vi "HandleObservationSync.vi"(8 "error in (no error)":errorcluster, 11 "S4GUI in":refnum<class "S4GUI.lvclass">) -> (0 "error out":errorcluster, 3 "S4GUI out":refnum<class "S4GUI.lvclass">)   [LabVIEW 2018, in "S4GUI.lvclass"] (continued)
            tunnel: w4132 -> [w4190 w4209]
            tunnel: [w4188 w4208] -> w4134
            tunnel: w4135 -> [w4189 _]
            tunnel: w4129 -> [w4187 _]
            frame False {
              n1517 = case shown="0, Default" w4187 {
                selector: w4187 -> [_ w4204]
                tunnel: [w4191 w4199] -> w4188
                tunnel: w4190 -> [w4194 w4205]
                tunnel: w4189 -> [w4193 _]
                frame 0, Default {
                  n1518 = disable-structure shown="Enabled" {
                    disable-tunnel: w4193 -> [w4196 w4197]
                    disable-tunnel: [w4195 w4197] -> w4192
                    frame Disabled {
                      # "Verifica o incremento \ndo CyclesDone simultaneamente"
                      n1519 = Increment(x=w4196) -> (x+1=w4195:u32)
                    }
                    frame Enabled {
                      # "OV20241106:\nNão verifica mais o CyclesDone\nem 327 enquanto espera o ACTIVE\nem 326."
                    }
                  }
                  n1520 = Bundle By Name(cluster=w4194, "Obs_state"=w4192) -> (w4191:refnum<class "S4GUI.lvclass">)
                }
                frame 1..15 {
                  n1521 = Number To Decimal String(number=w4204) -> (decimal integer string=w4201:string)  [unwired: 1 in]
                  n1522 = Concatenate Strings("CHANNEL ERROR <", w4201, ">: Error flag TRUE - see ACS panel.  HandleObservationSync.vi - state 326.") -> (w4203:string)
                  n1523 = Bundle By Name(cluster=w4205, "Obs_state"=u32 1, "Error Msg"=w4203) -> (w4199:refnum<class "S4GUI.lvclass">)
                }
              }
            }
            frame True {
              # "ACTIVE detectado.\nIniciou aquisição..."
              n1524 = Tick Count (ms)() -> (millisecond timer value=w4206:u32)
              n1525 = local write "time307"(w4206) -> ()
              n1526 = Bundle By Name(cluster=w4209, "Obs_state"=u32 328) -> (w4208:refnum<class "S4GUI.lvclass">)
            }
          }
          n1527 = Bundle By Name(cluster=w4134, "mode EXPOSE"=w4137) -> (w4181:refnum<class "S4GUI.lvclass">)
        }
        frame 327 {
          # "T= canais receberam STOP"
          n1528 = Unbundle By Name(w4333) -> ("cyclesDone"=w4328:u32)
          n1529 = call-dynamic "Read AcquisitionA.vi"("error in (no error)"=w4366, "S4ACS_GUI in"=w4333) -> ("error out"=w4348:errorcluster, "Acquisition.lvclass"=w4349:refnum<class "Acquisition.lvclass">, "S4ACS_GUI out"=w4368:refnum<class "S4GUI.lvclass">)  [unwired: 7 in]
          n1530 = call-dynamic "Read enabled.vi"("error in (no error)"=w4348, "Server in"=w4349) -> ("error out"=w4347:errorcluster, "enabled"=w4324:bool, "Server out"=w4346:refnum<class "Acquisition.lvclass">)  [unwired: 7 in]
          n1531 = case shown="True" w4324 {
            tunnel: w4347 -> [w4522 w4539]
            tunnel: [w4523 w4537] -> w4369
            tunnel: [w4522 w4536] -> w4367
            tunnel: [0 ("State") w4532] -> w4319
            tunnel: w4346 -> [w4523 w4531]
            tunnel: w4328 -> [_ w4530]
            tunnel: [TRUE w4529] -> w4332
            tunnel: [FALSE ("stopping") w4525] -> w4315
            frame False {
            }
            frame True {
              n1532 = call-dynamic "Read Channel.vi"("error in (no error)"=w4539, "Acquisition in"=w4531) -> ("error out"=w4535:errorcluster, "Channel.lvclass"=w4534:refnum<class "Channel.lvclass">, "Acquisition out"=w4538:refnum<class "Acquisition.lvclass">)  [unwired: 7 in]
              n1533 = call-dynamic "Read CyclesDone.vi"("error in (no error)"=w4535, "Channel in"=w4534) -> ("error out"=w4527:errorcluster, "CyclesDone"=w4532:u32, "Channel out"=w4533:refnum<class "Channel.lvclass">)  [unwired: 7 in]
              n1534 = Increment(x=w4530) -> (x+1=w4524:u32)
              n1535 = Equal?(x=w4532, y=w4524) -> (x = y?=w4529:bool)
              n1536 = call-dynamic "Read stopping.vi"("error in (no error)"=w4527, "Channel in"=w4533) -> ("error out"=w4526:errorcluster, "stopping"=w4525:bool, "Channel out"=w4528:refnum<class "Channel.lvclass">)  [unwired: 7 in]
              n1537 = call-dynamic "Write Channel.vi"("error in (no error)"=w4526, "Channel.lvclass"=w4528, "Acquisition in"=w4538) -> ("error out"=w4536:errorcluster, "Acquisition out"=w4537:refnum<class "Acquisition.lvclass">)  [unwired: 7 in]
            }
          }
          n1538 = call-dynamic "Write AcquisitionA.vi"("error in (no error)"=w4367, "Acquisition.lvclass"=w4369, "S4ACS_GUI in"=w4368) -> ("error out"=w4364:errorcluster, "S4ACS_GUI out"=w4363:refnum<class "S4GUI.lvclass">)  [unwired: 7 in]
          n1539 = call "Read AcquisitionB.vi"("error in (no error)"=w4364, "S4ACS_GUI in"=w4363) -> ("error out"=w4342:errorcluster, "Acquisition.lvclass"=w4345:refnum<class "Acquisition.lvclass">, "S4ACS_GUI out"=w4365:refnum<class "S4GUI.lvclass">)  [unwired: 7 in]
          n1540 = call-dynamic "Read enabled.vi"("error in (no error)"=w4342, "Server in"=w4345) -> ("error out"=w4343:errorcluster, "enabled"=w4323:bool, "Server out"=w4344:refnum<class "Acquisition.lvclass">)  [unwired: 7 in]
          n1541 = case shown="True" w4323 {
            tunnel: w4343 -> [w4501 w4518]
            tunnel: w4344 -> [w4502 w4517]
            tunnel: [0 ("State") w4510] -> w4318
            tunnel: [w4501 w4516] -> w4362
            tunnel: [w4502 w4515] -> w4361
            tunnel: w4328 -> [_ w4509]
            tunnel: [TRUE w4508] -> w4329
            tunnel: [FALSE ("stopping") w4504] -> w4314
            frame False {
            }
            frame True {
              n1542 = call-dynamic "Read Channel.vi"("error in (no error)"=w4518, "Acquisition in"=w4517) -> ("error out"=w4513:errorcluster, "Channel.lvclass"=w4514:refnum<class "Channel.lvclass">, "Acquisition out"=w4511:refnum<class "Acquisition.lvclass">)  [unwired: 7 in]
              n1543 = call-dynamic "Read CyclesDone.vi"("error in (no error)"=w4513, "Channel in"=w4514) -> ("error out"=w4506:errorcluster, "CyclesDone"=w4510:u32, "Channel out"=w4512:refnum<class "Channel.lvclass">)  [unwired: 7 in]
              n1544 = Increment(x=w4509) -> (x+1=w4503:u32)
              n1545 = Equal?(x=w4510, y=w4503) -> (x = y?=w4508:bool)
              n1546 = call-dynamic "Read stopping.vi"("error in (no error)"=w4506, "Channel in"=w4512) -> ("error out"=w4505:errorcluster, "stopping"=w4504:bool, "Channel out"=w4507:refnum<class "Channel.lvclass">)  [unwired: 7 in]
              n1547 = call-dynamic "Write Channel.vi"("error in (no error)"=w4505, "Channel.lvclass"=w4507, "Acquisition in"=w4511) -> ("error out"=w4516:errorcluster, "Acquisition out"=w4515:refnum<class "Acquisition.lvclass">)  [unwired: 7 in]
            }
          }
          n1548 = Max & Min(x=w4319, y=w4318) -> (max(x,y)=w4331:u32)  [unwired: 1 out]
          n1549 = call "Write AcquisitionB.vi"("error in (no error)"=w4362, "Acquisition.lvclass"=w4361, "S4ACS_GUI in"=w4365) -> ("error out"=w4354:errorcluster, "S4ACS_GUI out"=w4353:refnum<class "S4GUI.lvclass">)  [unwired: 7 in]
          n1550 = call-dynamic "Read AcquisitionC.vi"("error in (no error)"=w4354, "S4ACS_GUI in"=w4353) -> ("error out"=w4339:errorcluster, "Acquisition.lvclass"=w4341:refnum<class "Acquisition.lvclass">, "S4ACS_GUI out"=w4356:refnum<class "S4GUI.lvclass">)  [unwired: 7 in]
          n1551 = call-dynamic "Read enabled.vi"("error in (no error)"=w4339, "Server in"=w4341) -> ("error out"=w4338:errorcluster, "enabled"=w4322:bool, "Server out"=w4340:refnum<class "Acquisition.lvclass">)  [unwired: 7 in]
          n1552 = case shown="True" w4322 {
            tunnel: [w4480 w4497] -> w4357
            tunnel: [w4481 w4496] -> w4355
            tunnel: w4338 -> [w4480 w4493]
            tunnel: w4340 -> [w4481 w4494]
            tunnel: [0 ("State") w4492] -> w4317
            tunnel: w4328 -> [_ w4491]
            tunnel: [TRUE w4490] -> w4327
            tunnel: [FALSE ("stopping") w4483] -> w4313
            frame False {
            }
            frame True {
              n1553 = call-dynamic "Read Channel.vi"("error in (no error)"=w4493, "Acquisition in"=w4494) -> ("error out"=w4489:errorcluster, "Channel.lvclass"=w4488:refnum<class "Channel.lvclass">, "Acquisition out"=w4495:refnum<class "Acquisition.lvclass">)  [unwired: 7 in]
              n1554 = call-dynamic "Read CyclesDone.vi"("error in (no error)"=w4489, "Channel in"=w4488) -> ("error out"=w4485:errorcluster, "CyclesDone"=w4492:u32, "Channel out"=w4487:refnum<class "Channel.lvclass">)  [unwired: 7 in]
              n1555 = Increment(x=w4491) -> (x+1=w4482:u32)
              n1556 = Equal?(x=w4492, y=w4482) -> (x = y?=w4490:bool)
              n1557 = call-dynamic "Read stopping.vi"("error in (no error)"=w4485, "Channel in"=w4487) -> ("error out"=w4484:errorcluster, "stopping"=w4483:bool, "Channel out"=w4486:refnum<class "Channel.lvclass">)  [unwired: 7 in]
              n1558 = call-dynamic "Write Channel.vi"("error in (no error)"=w4484, "Channel.lvclass"=w4486, "Acquisition in"=w4495) -> ("error out"=w4497:errorcluster, "Acquisition out"=w4496:refnum<class "Acquisition.lvclass">)  [unwired: 7 in]
            }
          }
          n1559 = call-dynamic "Write AcquisitionC.vi"("error in (no error)"=w4357, "Acquisition.lvclass"=w4355, "S4ACS_GUI in"=w4356) -> ("error out"=w4351:errorcluster, "S4ACS_GUI out"=w4352:refnum<class "S4GUI.lvclass">)  [unwired: 7 in]
          n1560 = call-dynamic "Read AcquisitionD.vi"("error in (no error)"=w4351, "S4ACS_GUI in"=w4352) -> ("error out"=w4335:errorcluster, "Acquisition.lvclass"=w4337:refnum<class "Acquisition.lvclass">, "S4ACS_GUI out"=w4358:refnum<class "S4GUI.lvclass">)  [unwired: 7 in]
          n1561 = call-dynamic "Read enabled.vi"("error in (no error)"=w4335, "Server in"=w4337) -> ("error out"=w4334:errorcluster, "enabled"=w4325:bool, "Server out"=w4336:refnum<class "Acquisition.lvclass">)  [unwired: 7 in]
          n1562 = case shown="True" w4325 {
            tunnel: [w4460 w4476] -> w4360
            tunnel: [w4459 w4475] -> w4359
            tunnel: w4336 -> [w4460 w4474]
            tunnel: w4334 -> [w4459 w4473]
            tunnel: [0 ("State") w4471] -> w4316
            tunnel: w4328 -> [_ w4470]
            tunnel: [TRUE w4469] -> w4326
            tunnel: [FALSE ("stopping") w4462] -> w4312
            frame False {
            }
            frame True {
              n1563 = call-dynamic "Read Channel.vi"("error in (no error)"=w4473, "Acquisition in"=w4474) -> ("error out"=w4468:errorcluster, "Channel.lvclass"=w4467:refnum<class "Channel.lvclass">, "Acquisition out"=w4472:refnum<class "Acquisition.lvclass">)  [unwired: 7 in]
              n1564 = call-dynamic "Read CyclesDone.vi"("error in (no error)"=w4468, "Channel in"=w4467) -> ("error out"=w4464:errorcluster, "CyclesDone"=w4471:u32, "Channel out"=w4466:refnum<class "Channel.lvclass">)  [unwired: 7 in]
              n1565 = Increment(x=w4470) -> (x+1=w4461:u32)
              n1566 = Equal?(x=w4471, y=w4461) -> (x = y?=w4469:bool)
              n1567 = call-dynamic "Read stopping.vi"("error in (no error)"=w4464, "Channel in"=w4466) -> ("error out"=w4463:errorcluster, "stopping"=w4462:bool, "Channel out"=w4465:refnum<class "Channel.lvclass">)  [unwired: 7 in]
              n1568 = call-dynamic "Write Channel.vi"("error in (no error)"=w4463, "Channel.lvclass"=w4465, "Acquisition in"=w4472) -> ("error out"=w4475:errorcluster, "Acquisition out"=w4476:refnum<class "Acquisition.lvclass">)  [unwired: 7 in]
            }
          }
          n1569 = Build Array(w4324, w4323, w4322, w4325) -> (w4321:bool[])
          n1570 = Boolean Array To Number(Boolean array=w4321) -> (number=w4320:u32)
          n1571 = Max & Min(x=w4317, y=w4316) -> (max(x,y)=w4330:u32)  [unwired: 1 out]
          n1572 = Compound Arithmetic op=AND(w4332, w4329, w4327, w4326) -> (w4311:bool)
          n1573 = case shown="15" w4320 {
            tunnel: w4319 -> [w4412 _ w4424 _ w4433 _ w4439 w4445 _ w4451 w4454 _]
            tunnel: w4316 -> [w4411 w4415 w4420 w4427 w4428 w4436 w4438 _ _ _ _ _]
            tunnel: w4318 -> [w4410 w4413 _ _ w4432 w4434 _ w4444 w4448 _ w4453 _]
            tunnel: w4317 -> [w4409 w4414 w4419 w4425 _ _ _ w4443 w4447 w4450 _ _]
            tunnel: [w4405 w4416 w4421 w4426 w4429 w4435 w4437 w4440 w4446 w4449 w4452 TRUE] -> _
            frame 15 {
              # "A,B,C,D ativos"
              n1574 = Equal?(x=w4412, y=w4410) -> (x = y?=w4408:bool)
              n1575 = Equal?(x=w4409, y=w4411) -> (x = y?=w4406:bool)
              n1576 = Equal?(x=w4410, y=w4409) -> (x = y?=w4407:bool)
              n1577 = Compound Arithmetic op=AND(w4408, w4407, w4406) -> (w4405:bool)
            }
            frame 14 {
              # "B,C e,D ativos"
              n1578 = Equal?(x=w4413, y=w4414) -> (x = y?=w4418:bool)
              n1579 = Equal?(x=w4414, y=w4415) -> (x = y?=w4417:bool)
              n1580 = Compound Arithmetic op=AND(w4418, w4417) -> (w4416:bool)
            }
            frame 13 {
              # "A,C e,D ativos"
              n1581 = Equal?(x=w4424, y=w4419) -> (x = y?=w4423:bool)
              n1582 = Equal?(x=w4419, y=w4420) -> (x = y?=w4422:bool)
              n1583 = Compound Arithmetic op=AND(w4423, w4422) -> (w4421:bool)
            }
            frame 12 {
              # "Só C e D ativos"
              n1584 = Equal?(x=w4425, y=w4427) -> (x = y?=w4426:bool)
            }
            frame 11 {
              # "A,B e,D ativos"
              n1585 = Equal?(x=w4433, y=w4432) -> (x = y?=w4431:bool)
              n1586 = Equal?(x=w4432, y=w4428) -> (x = y?=w4430:bool)
              n1587 = Compound Arithmetic op=AND(w4431, w4430) -> (w4429:bool)
            }
            frame 10 {
              # "Só B e D ativos"
              n1588 = Equal?(x=w4434, y=w4436) -> (x = y?=w4435:bool)
            }
            frame 9 {
              # "Só A e D ativos"
              n1589 = Equal?(x=w4439, y=w4438) -> (x = y?=w4437:bool)
            }
            frame 7 {
              # "A,B,C ativos"
              n1590 = Equal?(x=w4445, y=w4444) -> (x = y?=w4442:bool)
              n1591 = Equal?(x=w4444, y=w4443) -> (x = y?=w4441:bool)
              n1592 = Compound Arithmetic op=AND(w4442, w4441) -> (w4440:bool)
            }
            frame 6 {
              # "Só B e C ativos"
              n1593 = Equal?(x=w4448, y=w4447) -> (x = y?=w4446:bool)
            }
            frame 5 {
              # "Só A e C ativos"
              n1594 = Equal?(x=w4451, y=w4450) -> (x = y?=w4449:bool)
            }
            frame 3 {
              # "só A e B ativos"
              n1595 = Equal?(x=w4454, y=w4453) -> (x = y?=w4452:bool)
            }
            frame 0..2, 4, 8, Default {
              # "nenhum ou só 1  \ncanal ativo."
            }
          }
          n1596 = Max & Min(x=w4331, y=w4330) -> (max(x,y)=w4309:u32)  [unwired: 1 out]
          n1597 = Compound Arithmetic op=OR(w4315, w4314, w4313, w4312) -> (w4310:bool)
          n1598 = call-dynamic "Write AcquisitionD.vi"("error in (no error)"=w4359, "Acquisition.lvclass"=w4360, "S4ACS_GUI in"=w4358) -> ("error out"=w4350:errorcluster, "S4ACS_GUI out"=w4307:refnum<class "S4GUI.lvclass">)  [unwired: 7 in]
          n1599 = case shown="False" w4311 {
            tunnel: w4307 -> [w4372 w4393]
            tunnel: [w4378 w4392] -> w4306
            tunnel: w4310 -> [_ w4394]
            tunnel: w4309 -> [_ w4391]
            tunnel: w4308 -> [w4370 w4390]
            frame False {
              # "Aguardando iniciar exposição por 5s"
              n1600 = local read "time1"() -> (w4371:u32)
              n1601 = Tick Count (ms)() -> (millisecond timer value=w4377:u32)
              n1602 = Subtract(x=w4377, y=w4371) -> (x-y=w4374:u32)
              n1603 = To Double Precision Float(number=w4374) -> (double precision float=w4376:dbl)
              n1604 = Less?(x=5000.0 ("y"), y=w4376) -> (x < y?=w4375:bool)
              n1605 = case shown="True" w4375 {
                tunnel: w4372 -> [w4382 w4389]
                tunnel: [w4381 w4388] -> w4378
                tunnel: w4370 -> [w4380 _]
                frame False {
                  n1606 = disable-structure shown="Enabled" {
                    disable-tunnel: w4380 -> [w4384 w4385]
                    disable-tunnel: [w4383 w4385] -> w4379
                    frame Disabled {
                      # "Volta para esperar ACTIVE."
                      n1607 = Decrement(x=w4384) -> (x-1=w4383:u32)
                    }
                    frame Enabled {
                    }
                  }
                  n1608 = Bundle By Name(cluster=w4382, "Obs_state"=w4379) -> (w4381:refnum<class "S4GUI.lvclass">)
                }
                frame True {
                  n1609 = Bundle By Name(cluster=w4389, "Obs_state"=u32 1, "Error Msg"="ERROR: Init Acquisition Timeout. HandleObservationSync.vi - state 327.") -> (w4388:refnum<class "S4GUI.lvclass">)
                }
              }
            }
            frame True {
              # "STOP?"
              # "CIclo Avançou."
              n1610 = case shown="False" w4394 {
                tunnel: w4393 -> [w4398 w4404]
                tunnel: [w4397 w4403] -> w4392
                tunnel: w4391 -> [w4396 w4402]
                tunnel: w4390 -> [_ w4401]
                frame True {
                  # "STOP acionado."
                  n1611 = Bundle By Name(cluster=w4398, "Obs_state"=u32 0, "cyclesDone"=w4396) -> (w4397:refnum<class "S4GUI.lvclass">)
                }
                frame False {
                  # "Vai verificar fim dos ciclos"
                  n1612 = Increment(x=w4401) -> (x+1=w4400:u32)
                  n1613 = Increment(x=w4400) -> (x+1=w4399:u32)
                  n1614 = Bundle By Name(cluster=w4404, "Obs_state"=w4399, "cyclesDone"=w4402) -> (w4403:refnum<class "S4GUI.lvclass">)
                }
              }
            }
          }
        }
        frame 328 {
          # "T= canais receberam STOP"
          n1615 = Unbundle By Name(w4564) -> ("cyclesDone"=w4558:u32)
          n1616 = call-dynamic "Read AcquisitionA.vi"("error in (no error)"=w4600, "S4ACS_GUI in"=w4564) -> ("error out"=w4579:errorcluster, "Acquisition.lvclass"=w4580:refnum<class "Acquisition.lvclass">, "S4ACS_GUI out"=w4602:refnum<class "S4GUI.lvclass">)  [unwired: 7 in]
          n1617 = call-dynamic "Read enabled.vi"("error in (no error)"=w4579, "Server in"=w4580) -> ("error out"=w4578:errorcluster, "enabled"=w4554:bool, "Server out"=w4577:refnum<class "Acquisition.lvclass">)  [unwired: 7 in]
          n1618 = case shown="False" w4554 {
            tunnel: w4578 -> [w4751 w4768]
            tunnel: [w4752 w4766] -> w4603
            tunnel: [w4751 w4765] -> w4601
            tunnel: [0 ("State") w4761] -> w4549
            tunnel: w4577 -> [w4752 w4760]
            tunnel: w4558 -> [_ w4759]
            tunnel: [TRUE w4758] -> w4563
            tunnel: [FALSE ("stopping") w4754] -> w4545
            frame False {
            }
            frame True {
              n1619 = call-dynamic "Read Channel.vi"("error in (no error)"=w4768, "Acquisition in"=w4760) -> ("error out"=w4764:errorcluster, "Channel.lvclass"=w4763:refnum<class "Channel.lvclass">, "Acquisition out"=w4767:refnum<class "Acquisition.lvclass">)  [unwired: 7 in]
              n1620 = call-dynamic "Read CyclesDone.vi"("error in (no error)"=w4764, "Channel in"=w4763) -> ("error out"=w4756:errorcluster, "CyclesDone"=w4761:u32, "Channel out"=w4762:refnum<class "Channel.lvclass">)  [unwired: 7 in]
              n1621 = Increment(x=w4759) -> (x+1=w4753:u32)
              n1622 = Equal?(x=w4761, y=w4753) -> (x = y?=w4758:bool)
              n1623 = call-dynamic "Read stopping.vi"("error in (no error)"=w4756, "Channel in"=w4762) -> ("error out"=w4755:errorcluster, "stopping"=w4754:bool, "Channel out"=w4757:refnum<class "Channel.lvclass">)  [unwired: 7 in]
              n1624 = call-dynamic "Write Channel.vi"("error in (no error)"=w4755, "Channel.lvclass"=w4757, "Acquisition in"=w4767) -> ("error out"=w4765:errorcluster, "Acquisition out"=w4766:refnum<class "Acquisition.lvclass">)  [unwired: 7 in]
            }
          }
          n1625 = call-dynamic "Write AcquisitionA.vi"("error in (no error)"=w4601, "Acquisition.lvclass"=w4603, "S4ACS_GUI in"=w4602) -> ("error out"=w4596:errorcluster, "S4ACS_GUI out"=w4595:refnum<class "S4GUI.lvclass">)  [unwired: 7 in]
          n1626 = call "Read AcquisitionB.vi"("error in (no error)"=w4596, "S4ACS_GUI in"=w4595) -> ("error out"=w4573:errorcluster, "Acquisition.lvclass"=w4576:refnum<class "Acquisition.lvclass">, "S4ACS_GUI out"=w4597:refnum<class "S4GUI.lvclass">)  [unwired: 7 in]
          n1627 = call-dynamic "Read enabled.vi"("error in (no error)"=w4573, "Server in"=w4576) -> ("error out"=w4574:errorcluster, "enabled"=w4553:bool, "Server out"=w4575:refnum<class "Acquisition.lvclass">)  [unwired: 7 in]
          n1628 = case shown="True" w4553 {
            tunnel: w4574 -> [w4730 w4747]
            tunnel: w4575 -> [w4731 w4746]
            tunnel: [0 ("State") w4739] -> w4548
            tunnel: [w4730 w4745] -> w4594
            tunnel: [w4731 w4744] -> w4593
            tunnel: w4558 -> [_ w4738]
            tunnel: [TRUE w4737] -> w4559
            tunnel: [FALSE ("stopping") w4733] -> w4544
            frame False {
            }
            frame True {
              n1629 = call-dynamic "Read Channel.vi"("error in (no error)"=w4747, "Acquisition in"=w4746) -> ("error out"=w4742:errorcluster, "Channel.lvclass"=w4743:refnum<class "Channel.lvclass">, "Acquisition out"=w4740:refnum<class "Acquisition.lvclass">)  [unwired: 7 in]
              n1630 = call-dynamic "Read CyclesDone.vi"("error in (no error)"=w4742, "Channel in"=w4743) -> ("error out"=w4735:errorcluster, "CyclesDone"=w4739:u32, "Channel out"=w4741:refnum<class "Channel.lvclass">)  [unwired: 7 in]
              n1631 = Increment(x=w4738) -> (x+1=w4732:u32)
              n1632 = Equal?(x=w4739, y=w4732) -> (x = y?=w4737:bool)
              n1633 = call-dynamic "Read stopping.vi"("error in (no error)"=w4735, "Channel in"=w4741) -> ("error out"=w4734:errorcluster, "stopping"=w4733:bool, "Channel out"=w4736:refnum<class "Channel.lvclass">)  [unwired: 7 in]
              n1634 = call-dynamic "Write Channel.vi"("error in (no error)"=w4734, "Channel.lvclass"=w4736, "Acquisition in"=w4740) -> ("error out"=w4745:errorcluster, "Acquisition out"=w4744:refnum<class "Acquisition.lvclass">)  [unwired: 7 in]
            }
          }
          n1635 = Max & Min(x=w4549, y=w4548) -> (max(x,y)=w4562:u32)  [unwired: 1 out]
          n1636 = call "Write AcquisitionB.vi"("error in (no error)"=w4594, "Acquisition.lvclass"=w4593, "S4ACS_GUI in"=w4597) -> ("error out"=w4586:errorcluster, "S4ACS_GUI out"=w4585:refnum<class "S4GUI.lvclass">)  [unwired: 7 in]
          n1637 = call-dynamic "Read AcquisitionC.vi"("error in (no error)"=w4586, "S4ACS_GUI in"=w4585) -> ("error out"=w4570:errorcluster, "Acquisition.lvclass"=w4572:refnum<class "Acquisition.lvclass">, "S4ACS_GUI out"=w4588:refnum<class "S4GUI.lvclass">)  [unwired: 7 in]
          n1638 = call-dynamic "Read enabled.vi"("error in (no error)"=w4570, "Server in"=w4572) -> ("error out"=w4569:errorcluster, "enabled"=w4552:bool, "Server out"=w4571:refnum<class "Acquisition.lvclass">)  [unwired: 7 in]
          n1639 = case shown="False" w4552 {
            tunnel: [w4709 w4726] -> w4589
            tunnel: [w4710 w4725] -> w4587
            tunnel: w4569 -> [w4709 w4722]
            tunnel: w4571 -> [w4710 w4723]
            tunnel: [0 ("State") w4721] -> w4547
            tunnel: w4558 -> [_ w4720]
            tunnel: [TRUE w4719] -> w4557
            tunnel: [FALSE ("stopping") w4712] -> w4543
            frame False {
            }
            frame True {
              n1640 = call-dynamic "Read Channel.vi"("error in (no error)"=w4722, "Acquisition in"=w4723) -> ("error out"=w4718:errorcluster, "Channel.lvclass"=w4717:refnum<class "Channel.lvclass">, "Acquisition out"=w4724:refnum<class "Acquisition.lvclass">)  [unwired: 7 in]
              n1641 = call-dynamic "Read CyclesDone.vi"("error in (no error)"=w4718, "Channel in"=w4717) -> ("error out"=w4714:errorcluster, "CyclesDone"=w4721:u32, "Channel out"=w4716:refnum<class "Channel.lvclass">)  [unwired: 7 in]
              n1642 = Increment(x=w4720) -> (x+1=w4711:u32)
              n1643 = Equal?(x=w4721, y=w4711) -> (x = y?=w4719:bool)
              n1644 = call-dynamic "Read stopping.vi"("error in (no error)"=w4714, "Channel in"=w4716) -> ("error out"=w4713:errorcluster, "stopping"=w4712:bool, "Channel out"=w4715:refnum<class "Channel.lvclass">)  [unwired: 7 in]
              n1645 = call-dynamic "Write Channel.vi"("error in (no error)"=w4713, "Channel.lvclass"=w4715, "Acquisition in"=w4724) -> ("error out"=w4726:errorcluster, "Acquisition out"=w4725:refnum<class "Acquisition.lvclass">)  [unwired: 7 in]
            }
          }
          n1646 = call-dynamic "Write AcquisitionC.vi"("error in (no error)"=w4589, "Acquisition.lvclass"=w4587, "S4ACS_GUI in"=w4588) -> ("error out"=w4583:errorcluster, "S4ACS_GUI out"=w4584:refnum<class "S4GUI.lvclass">)  [unwired: 7 in]
          n1647 = call-dynamic "Read AcquisitionD.vi"("error in (no error)"=w4583, "S4ACS_GUI in"=w4584) -> ("error out"=w4566:errorcluster, "Acquisition.lvclass"=w4568:refnum<class "Acquisition.lvclass">, "S4ACS_GUI out"=w4590:refnum<class "S4GUI.lvclass">)  [unwired: 7 in]
          n1648 = call-dynamic "Read enabled.vi"("error in (no error)"=w4566, "Server in"=w4568) -> ("error out"=w4565:errorcluster, "enabled"=w4555:bool, "Server out"=w4567:refnum<class "Acquisition.lvclass">)  [unwired: 7 in]
          n1649 = case shown="True" w4555 {
            tunnel: [w4689 w4705] -> w4592
            tunnel: [w4688 w4704] -> w4591
            tunnel: w4567 -> [w4689 w4703]
            tunnel: w4565 -> [w4688 w4702]
            tunnel: [0 ("State") w4700] -> w4546
            tunnel: w4558 -> [_ w4699]
            tunnel: [TRUE w4698] -> w4556
            tunnel: [FALSE ("stopping") w4691] -> w4542
            frame False {
            }
            frame True {
              n1650 = call-dynamic "Read Channel.vi"("error in (no error)"=w4702, "Acquisition in"=w4703) -> ("error out"=w4697:errorcluster, "Channel.lvclass"=w4696:refnum<class "Channel.lvclass">, "Acquisition out"=w4701:refnum<class "Acquisition.lvclass">)  [unwired: 7 in]
              n1651 = call-dynamic "Read CyclesDone.vi"("error in (no error)"=w4697, "Channel in"=w4696) -> ("error out"=w4693:errorcluster, "CyclesDone"=w4700:u32, "Channel out"=w4695:refnum<class "Channel.lvclass">)  [unwired: 7 in]
              n1652 = Increment(x=w4699) -> (x+1=w4690:u32)
              n1653 = Equal?(x=w4700, y=w4690) -> (x = y?=w4698:bool)
              n1654 = call-dynamic "Read stopping.vi"("error in (no error)"=w4693, "Channel in"=w4695) -> ("error out"=w4692:errorcluster, "stopping"=w4691:bool, "Channel out"=w4694:refnum<class "Channel.lvclass">)  [unwired: 7 in]
              n1655 = call-dynamic "Write Channel.vi"("error in (no error)"=w4692, "Channel.lvclass"=w4694, "Acquisition in"=w4701) -> ("error out"=w4704:errorcluster, "Acquisition out"=w4705:refnum<class "Acquisition.lvclass">)  [unwired: 7 in]
            }
          }
          n1656 = Build Array(w4554, w4553, w4552, w4555) -> (w4551:bool[])
          n1657 = Boolean Array To Number(Boolean array=w4551) -> (number=w4550:u32)
          n1658 = Max & Min(x=w4547, y=w4546) -> (max(x,y)=w4561:u32)  [unwired: 1 out]
          n1659 = Compound Arithmetic op=AND(w4563, w4559, w4557, w4556) -> (w4540:bool)
          n1660 = case shown="15" w4550 {
            tunnel: w4549 -> [w4611 _ w4623 _ w4632 _ w4638 w4644 _ w4650 w4653 _]
            tunnel: w4546 -> [w4610 w4614 w4619 w4626 w4627 w4635 w4637 _ _ _ _ _]
            tunnel: w4548 -> [w4609 w4612 _ _ w4631 w4633 _ w4643 w4647 _ w4652 _]
            tunnel: w4547 -> [w4608 w4613 w4618 w4624 _ _ _ w4642 w4646 w4649 _ _]
            tunnel: [w4604 w4615 w4620 w4625 w4628 w4634 w4636 w4639 w4645 w4648 w4651 TRUE] -> _
            frame 15 {
              # "A,B,C,D ativos"
              n1661 = Equal?(x=w4611, y=w4609) -> (x = y?=w4607:bool)
              n1662 = Equal?(x=w4608, y=w4610) -> (x = y?=w4605:bool)
              n1663 = Equal?(x=w4609, y=w4608) -> (x = y?=w4606:bool)
              n1664 = Compound Arithmetic op=AND(w4607, w4606, w4605) -> (w4604:bool)
            }
            frame 14 {
              # "B,C e,D ativos"
              n1665 = Equal?(x=w4612, y=w4613) -> (x = y?=w4617:bool)
              n1666 = Equal?(x=w4613, y=w4614) -> (x = y?=w4616:bool)
              n1667 = Compound Arithmetic op=AND(w4617, w4616) -> (w4615:bool)
            }
            frame 13 {
              # "A,C e,D ativos"
              n1668 = Equal?(x=w4623, y=w4618) -> (x = y?=w4622:bool)
              n1669 = Equal?(x=w4618, y=w4619) -> (x = y?=w4621:bool)
              n1670 = Compound Arithmetic op=AND(w4622, w4621) -> (w4620:bool)
            }
            frame 12 {
              # "Só C e D ativos"
              n1671 = Equal?(x=w4624, y=w4626) -> (x = y?=w4625:bool)
            }
            frame 11 {
              # "A,B e,D ativos"
              n1672 = Equal?(x=w4632, y=w4631) -> (x = y?=w4630:bool)
              n1673 = Equal?(x=w4631, y=w4627) -> (x = y?=w4629:bool)
              n1674 = Compound Arithmetic op=AND(w4630, w4629) -> (w4628:bool)
            }
            frame 10 {
              # "Só B e D ativos"
              n1675 = Equal?(x=w4633, y=w4635) -> (x = y?=w4634:bool)
            }
            frame 9 {
              # "Só A e D ativos"
              n1676 = Equal?(x=w4638, y=w4637) -> (x = y?=w4636:bool)
            }
            frame 7 {
              # "A,B,C ativos"
              n1677 = Equal?(x=w4644, y=w4643) -> (x = y?=w4641:bool)
              n1678 = Equal?(x=w4643, y=w4642) -> (x = y?=w4640:bool)
              n1679 = Compound Arithmetic op=AND(w4641, w4640) -> (w4639:bool)
            }
            frame 6 {
              # "Só B e C ativos"
              n1680 = Equal?(x=w4647, y=w4646) -> (x = y?=w4645:bool)
            }
            frame 5 {
              # "Só A e C ativos"
              n1681 = Equal?(x=w4650, y=w4649) -> (x = y?=w4648:bool)
            }
            frame 3 {
              # "só A e B ativos"
              n1682 = Equal?(x=w4653, y=w4652) -> (x = y?=w4651:bool)
            }
            frame 0..2, 4, 8, Default {
              # "nenhum ou só 1  \ncanal ativo."
            }
          }
          n1683 = Max & Min(x=w4562, y=w4561) -> (max(x,y)=w4560:u32)  [unwired: 1 out]
          n1684 = Compound Arithmetic op=OR(w4545, w4544, w4543, w4542) -> (w4541:bool)
          n1685 = call-dynamic "Write AcquisitionD.vi"("error in (no error)"=w4591, "Acquisition.lvclass"=w4592, "S4ACS_GUI in"=w4590) -> ("error out"=w4581:errorcluster, "S4ACS_GUI out"=w4582:refnum<class "S4GUI.lvclass">)  [unwired: 7 in]
          n1686 = case shown="False" w4540 {
            tunnel: w4582 -> [w4665 w4675]
            tunnel: [w4664 w4674] -> w4599
            tunnel: w4598 -> [_ w4673]
            tunnel: w4560 -> [_ w4672]
            tunnel: w4541 -> [_ w4671]
            frame False {
              # "Aguardando avanço do ciclo."
              n1687 = local read "time307"() -> (w4655:u32)
              n1688 = Tick Count (ms)() -> (millisecond timer value=w4663:u32)
              n1689 = Subtract(x=w4663, y=w4655) -> (x-y=w4660:u32)
              n1690 = call-dynamic "GetGreatestCube.vi"("S4GUI in"=w4665) -> ("S4GUI out"=w4656:refnum<class "S4GUI.lvclass">, "greatest (ms)"=w4658:dbl)  [unwired: 8 in, 1 out]
              n1691 = To Double Precision Float(number=w4660) -> (double precision float=w4662:dbl)
              n1692 = Add(x=5000.0 ("y"), y=w4658) -> (x+y=w4657:dbl)
              n1693 = Less?(x=w4657, y=w4662) -> (x < y?=w4661:bool)
              n1694 = case shown="False" w4661 {
                tunnel: w4656 -> [w4666 w4670]
                tunnel: [w4666 w4669] -> w4664
                frame False {
                }
                frame True {
                  n1695 = Bundle By Name(cluster=w4670, "Obs_state"=u32 1, "Error Msg"="ERROR: Acquisition Timeout. HandleObservationSync.vi - state 328.") -> (w4669:refnum<class "S4GUI.lvclass">)
                }
              }
            }
            frame True {
              # "Ciclo avançou."
              # "STOP?"
              n1696 = case shown="False" w4671 {
                tunnel: w4675 -> [w4679 w4684]
                tunnel: [w4678 w4683] -> w4674
                tunnel: w4673 -> [_ w4681]
                tunnel: w4672 -> [w4677 w4680]
                frame True {
                  n1697 = Bundle By Name(cluster=w4679, "Obs_state"=u32 0, "cyclesDone"=w4677) -> (w4678:refnum<class "S4GUI.lvclass">)
                }
                frame False {
                  n1698 = Increment(x=w4681) -> (x+1=w4682:u32)
                  n1699 = Bundle By Name(cluster=w4684, "Obs_state"=w4682, "cyclesDone"=w4680) -> (w4683:refnum<class "S4GUI.lvclass">)
                }
              }
            }
          }
        }
        frame 329 {
          n1700 = disable-structure shown="Enabled" {
            disable-tunnel: w4773 -> [w4787 w4793]
            disable-tunnel: w4772 -> [w4786 w4800]
            disable-tunnel: [w4785 w4800] -> w4771
            disable-tunnel: [w4783 w4801] -> w4770
            disable-tunnel: w4769 -> [_ w4794]
            frame Disabled {
              n1701 = call-dynamic "Read ciclos.vi"("error in (no error)"=w4786, "S4ACS_GUI in"=w4787) -> ("error out"=w4775:errorcluster, "ciclos"=w4780:u32, "S4ACS_GUI out"=w4788:refnum<class "S4GUI.lvclass">)  [unwired: 7 in]
              n1702 = Decrement(x=w4780) -> (x-1=w4774:u32)
              n1703 = Greater Than 0?(x=w4774) -> (x > 0?=w4781:bool)
              n1704 = case shown="False" w4781 {
                selector: w4781 -> [w4790 w4792]
                tunnel: w4774 -> [_ w4791]
                tunnel: [w4790 w4792] -> w4779
                tunnel: [u32 0 w4791] -> w4776
                frame False {
                }
                frame True {
                }
              }
              n1705 = Select(t=u32 323, s=w4779, f=u32 0) -> (s? t:f=w4782:u32)
              n1706 = call-dynamic "Write ciclos.vi"("error in (no error)"=w4775, "ciclos"=w4776, "S4ACS_GUI in"=w4788) -> ("error out"=w4785:errorcluster, "S4ACS_GUI out"=w4784:refnum<class "S4GUI.lvclass">)  [unwired: 7 in]
              n1707 = Bundle By Name(cluster=w4784, "Obs_state"=w4782) -> (w4783:refnum<class "S4GUI.lvclass">)
            }
            frame Enabled {
              n1708 = Unbundle By Name(w4793) -> ("TotalCiclos"=w4803:u32, "cyclesDone"=w4802:u32)
              n1709 = Subtract(x=w4803, y=w4802) -> (x-y=w4796:u32)
              n1710 = Greater Than 0?(x=w4796) -> (x > 0?=w4799:bool)
              n1711 = disable-structure shown="Enabled" {
                disable-tunnel: [w4805 u32 325 ("t")] -> w4795
                disable-tunnel: w4794 -> [w4804 _]
                frame Disabled {
                  n1712 = Increment(x=w4804) -> (x+1=w4805:u32)
                }
                frame Enabled {
                }
              }
              n1713 = Select(t=w4795, s=w4799, f=u32 0) -> (s? t:f=w4798:u32)
              n1714 = Bundle By Name(cluster=w4793, "ciclos"=w4796, "Obs_state"=w4798) -> (w4801:refnum<class "S4GUI.lvclass">)
            }
          }
        }
        frame 350 {
          n1715 = flat-sequence {
            tunnel: w4808 -> [w4848]
            tunnel: [w4848] -> w4807
            frame #0 {
              n1716 = Tick Count (ms)() -> (millisecond timer value=→"timer350":u32)
            }
          }
          n1717 = call "Read Instrument.lvclass.vi"("error in (no error)"=w4807, "S4ACS_GUI in"=w4843) -> ("error out"=w4846:errorcluster, "Instrument.lvclass"=w4847:refnum<class "Instrument.lvclass">, "S4ACS_GUI out"=w4844:refnum<class "S4GUI.lvclass">)  [unwired: 7 in]
          n1718 = call "Read WPROT.vi"("error in (no error)"=w4846, "Instrument in"=w4847) -> ("error out"=w4836:errorcluster, "Opt_Selector.lvclass"=w4837:refnum<class "Opt_Selector.lvclass">, "Instrument out"=w4845:refnum<class "Instrument.lvclass">)  [unwired: 7 in]
          n1719 = call-dynamic "getTargetPos.vi"("error in (no error)"=w4836, "Opt_Selector in"=w4837) -> ("error out"=w4835:errorcluster, "Target Pos"=w4815:u16, "Opt_Selector out"=w4834:refnum<class "Opt_Selector.lvclass">)  [unwired: 7 in]
          n1720 = Build Array(-1.0 ("element"), 0.0 ("element"), 22.5 ("element"), 45.0 ("element"), 67.5 ("element"), 90.0 ("element"), 112.5 ("element"), 135.0 ("element"), 157.5 ("element"), 180.0 ("element"), 202.5 ("element"), 225.0 ("element"), 247.5 ("element"), 270.0 ("element"), 292.5 ("element"), 315.0 ("element"), 337.5 ("element")) -> (w4827:dbl[])
          n1721 = Index Array(array=w4827, index=w4815) -> (element=w4814:dbl)
          n1722 = case shown="0, Default" w4815 {
            selector: w4815 -> [_ w4877]
            tunnel: w4845 -> [w4857 w4865]
            tunnel: [w4857 w4865] -> w4810
            tunnel: [w4854 w4864] -> w4809
            tunnel: w4840 -> [_ w4879]
            tunnel: [u32 352 w4878] -> w4839
            tunnel: w4835 -> [w4855 w4873]
            tunnel: w4834 -> [w4856 w4872]
            tunnel: w4814 -> [_ w4867]
            tunnel: [w4852 w4866] -> w4811
            frame 0, Default {
              # "Terminou uma sequência.\nRecupera as posições em SEQ e desvia para 311 para verificar se há mais ciclos."
              # "Recupera a sequencia anterior para o caso \nde repetição da sequencia (sem precisar clicar \nnas posicoes desejadas novamente)."
              n1723 = call-dynamic "Read sequencia_ant.vi"("error in (no error)"=w4855, "Opt_Selector in"=w4856) -> ("error out"=w4851:errorcluster, "sequencia_ant"=w4850:u16, "Opt_Selector out"=w4853:refnum<class "Opt_Selector.lvclass">)  [unwired: 7 in]
              n1724 = call-dynamic "Write sequencia.vi"("error in (no error)"=w4851, "sequencia"=w4850, "Opt_Selector in"=w4853) -> ("error out"=w4854:errorcluster, "Opt_Selector out"=w4852:refnum<class "Opt_Selector.lvclass">)  [unwired: 7 in]
            }
            frame 1..16 {
              # "Espera até 40 x 0.25s (= 10s) para\nmecanismo entrar em READY"
              n1725 = Number To Decimal String(number=w4877) -> (decimal integer string=w4876:string)  [unwired: 1 in]
              n1726 = Concatenate Strings("WP" ("string"), w4876) -> (w4874:string)
              n1727 = call "Write target name.vi"("error in (no error)"=w4873, "target name"=w4874, "Optics in"=w4872) -> ("error out"=w4870:errorcluster, "Optics out"=w4871:refnum<class "Opt_Selector.lvclass">)  [unwired: 7 in]
              n1728 = call "Write target.vi"("error in (no error)"=w4870, "target"=w4867, "Optics in"=w4871) -> ("error out"=w4869:errorcluster, "Optics out"=w4868:refnum<class "Opt_Selector.lvclass">)  [unwired: 7 in]
              n1729 = call-dynamic "Read State Machine.vi"("error in (no error)"=w4869, "Device in"=w4868) -> ("error out"=w4881:errorcluster, "State Machine.lvclass"=w4883:refnum<class "State Machine.lvclass">, "Device out"=w4880:refnum<class "Opt_Selector.lvclass">)  [unwired: 7 in]
              n1730 = Increment(x=w4879) -> (x+1=w4878:u32)
              n1731 = call "Next State.vi"("error in (no error)"=w4881, "New_State"=1, "State Machine in"=w4883) -> ("error out"=w4861:errorcluster, "State Machine out"=w4863:refnum<class "State Machine.lvclass">)  [unwired: 7 in]
              n1732 = call-dynamic "Write Timer.vi"("error in (no error)"=w4861, "Timer"=u32 40, "State Machine in"=w4863) -> ("error out"=w4860:errorcluster, "State Machine out"=w4862:refnum<class "State Machine.lvclass">)  [unwired: 7 in]
              n1733 = call-dynamic "Write State Machine.vi"("error in (no error)"=w4860, "State Machine.lvclass"=w4862, "Device in"=w4880) -> ("error out"=w4864:errorcluster, "Device out"=w4866:refnum<class "Opt_Selector.lvclass">)  [unwired: 7 in]
            }
          }
          n1734 = call "Write WPROT.vi"("error in (no error)"=w4809, "Opt_Selector.lvclass"=w4811, "Instrument in"=w4810) -> ("error out"=w4813:errorcluster, "Instrument out"=w4812:refnum<class "Instrument.lvclass">)  [unwired: 7 in]
          n1735 = call "Write Instrument.lvclass.vi"("error in (no error)"=w4813, "Instrument.lvclass"=w4812, "S4ACS_GUI in"=w4844) -> ("error out"=w4842:errorcluster, "S4ACS_GUI out"=w4841:refnum<class "S4GUI.lvclass">)  [unwired: 7 in]
          n1736 = Bundle By Name(cluster=w4841, "Obs_state"=w4839) -> (w4838:refnum<class "S4GUI.lvclass">)
        }
        frame 351 {
          # "Espera terminar o movimento da lamina para disparar a aquisição\ndos canais ativos.\n\nOV 20230424: Não precisa mais atualizar o valor de WPPOS com o\ncomando WRITE_HEADER porque o ACS já recebeu a sequência de\nposições da lâmina."
          n1737 = flat-sequence {
            tunnel: w4894 -> [w4913]
            tunnel: [w4913] -> w4893
            frame #0 {
              n1738 = Tick Count (ms)() -> (millisecond timer value=w4912:u32)
              "timer351" <- w4912
              n1739 = local read "time1"() -> (w4911:u32)
              n1740 = Subtract(x=w4912, y=w4911) -> (x-y=→"delay wp 2":u32)
            }
          }
          n1741 = call "Read Instrument.lvclass.vi"("error in (no error)"=w4893, "S4ACS_GUI in"=w4903) -> ("error out"=w4908:errorcluster, "Instrument.lvclass"=w4909:refnum<class "Instrument.lvclass">, "S4ACS_GUI out"=w4905:refnum<class "S4GUI.lvclass">)  [unwired: 7 in]
          n1742 = call "Read WPROT.vi"("error in (no error)"=w4908, "Instrument in"=w4909) -> ("error out"=w4900:errorcluster, "Opt_Selector.lvclass"=w4899:refnum<class "Opt_Selector.lvclass">, "Instrument out"=w4907:refnum<class "Instrument.lvclass">)  [unwired: 7 in]
          n1743 = call-dynamic "Read State Machine.vi"("error in (no error)"=w4900, "Device in"=w4899) -> ("error out"=w4901:errorcluster, "State Machine.lvclass"=w4902:refnum<class "State Machine.lvclass">, "Device out"=w4897:refnum<class "Opt_Selector.lvclass">)  [unwired: 7 in]
          n1744 = call-dynamic "Read State.vi"("error in (no error)"=w4901, "State Machine in"=w4902) -> ("error out"=w4891:errorcluster, "State"=w4895:i32, "State Machine out"=w4892:refnum<class "State Machine.lvclass">)  [unwired: 7 in]
          n1745 = Equal To 0?(x=w4895) -> (x = 0?=w4886:bool)
          n1746 = call-dynamic "Write State Machine.vi"("error in (no error)"=w4891, "State Machine.lvclass"=w4892, "Device in"=w4897) -> ("error out"=w4896:errorcluster, "Device out"=w4898:refnum<class "Opt_Selector.lvclass">)  [unwired: 7 in]
          n1747 = call "Write WPROT.vi"("error in (no error)"=w4896, "Opt_Selector.lvclass"=w4898, "Instrument in"=w4907) -> ("error out"=w4904:errorcluster, "Instrument out"=w4906:refnum<class "Instrument.lvclass">)  [unwired: 7 in]
          n1748 = call "Write Instrument.lvclass.vi"("error in (no error)"=w4904, "Instrument.lvclass"=w4906, "S4ACS_GUI in"=w4905) -> ("error out"=w4884:errorcluster, "S4ACS_GUI out"=w4887:refnum<class "S4GUI.lvclass">)  [unwired: 7 in]
          n1749 = Select(t=u32 350, s=w4886, f=w4885) -> (s? t:f=w4890:u32)
          n1750 = Bundle By Name(cluster=w4887, "Obs_state"=w4890) -> (w4888:refnum<class "S4GUI.lvclass">)
        }
        frame 352 {
          n1751 = disable-structure shown="Enabled" {
            disable-tunnel: w4917 -> [w4931 w4944]
            disable-tunnel: w4916 -> [w4930 w4942]
            disable-tunnel: [w4929 w4942] -> w4915
            disable-tunnel: [w4927 w4943] -> w4914
            frame Disabled {
              n1752 = call-dynamic "Read ciclos.vi"("error in (no error)"=w4930, "S4ACS_GUI in"=w4931) -> ("error out"=w4919:errorcluster, "ciclos"=w4924:u32, "S4ACS_GUI out"=w4932:refnum<class "S4GUI.lvclass">)  [unwired: 7 in]
              n1753 = Decrement(x=w4924) -> (x-1=w4918:u32)
              n1754 = Greater Than 0?(x=w4918) -> (x > 0?=w4925:bool)
              n1755 = case shown="False" w4925 {
                selector: w4925 -> [w4934 w4936]
                tunnel: w4918 -> [_ w4935]
                tunnel: [w4934 w4936] -> w4923
                tunnel: [u32 0 w4935] -> w4920
                frame False {
                }
                frame True {
                }
              }
              n1756 = Select(t=u32 323, s=w4923, f=u32 0) -> (s? t:f=w4926:u32)
              n1757 = call-dynamic "Write ciclos.vi"("error in (no error)"=w4919, "ciclos"=w4920, "S4ACS_GUI in"=w4932) -> ("error out"=w4929:errorcluster, "S4ACS_GUI out"=w4928:refnum<class "S4GUI.lvclass">)  [unwired: 7 in]
              n1758 = Bundle By Name(cluster=w4928, "Obs_state"=w4926) -> (w4927:refnum<class "S4GUI.lvclass">)
            }
            frame Enabled {
              n1759 = Unbundle By Name(w4944) -> ("cycles wprot"=w4945:u32)
              n1760 = Decrement(x=w4945) -> (x-1=w4937:u32)
              n1761 = Greater Than 0?(x=w4937) -> (x > 0?=w4941:bool)
              n1762 = Select(t=u32 350, s=w4941, f=u32 0) -> (s? t:f=w4940:u32)
              n1763 = Bundle By Name(cluster=w4944, "Obs_state"=w4940, "cycles wprot"=w4937) -> (w4943:refnum<class "S4GUI.lvclass">)
            }
          }
        }
        frame 360 {
          w4946 = u32 0 ("cyclesDone")
          # "Inicia o Ticks com\nvalor do relogio atual"
          # "Espera até 40 x 0.25s (= 10s) para\nmecanismo entrar em READY"
          # "Busca próximo valor de foco..."
          n1764 = flat-sequence {
            tunnel: w4963 -> [w4978]
            tunnel: [w4978] -> w4962
            frame #0 {
              n1765 = Tick Count (ms)() -> (millisecond timer value=→"time7":u32)
            }
          }
          n1766 = call-dynamic "Read TelFocus.lvclass.vi"("error in (no error)"=w4962, "S4GUI in"=w4974) -> ("error out"=w4976:errorcluster, "TelFocus.lvclass"=w4977:refnum<class "TelFocus.lvclass">, "S4GUI out"=w4975:refnum<class "S4GUI.lvclass">)  [unwired: 7 in]
          n1767 = call-dynamic "GetNextFocus.vi"("error in (no error)"=w4976, "TelFocus in"=w4977) -> ("error out"=w4960:errorcluster, "TelFocus out"=w4961:refnum<class "TelFocus.lvclass">)  [unwired: 8 in]
          n1768 = call-dynamic "Read SecMirror.lvclass.vi"("error in (no error)"=w4960, "TelFocus in"=w4961) -> ("error out"=w4947:errorcluster, "SecMirror.lvclass"=w4948:refnum<class "SecMirror.lvclass">, "TelFocus out"=w4965:refnum<class "TelFocus.lvclass">)  [unwired: 7 in]
          n1769 = call-dynamic "Read State Machine.vi"("error in (no error)"=w4947, "Device in"=w4948) -> ("error out"=w4957:errorcluster, "State Machine.lvclass"=w4959:refnum<class "State Machine.lvclass">, "Device out"=w4956:refnum<class "SecMirror.lvclass">)  [unwired: 7 in]
          n1770 = call "Next State.vi"("error in (no error)"=w4957, "New_State"=1, "State Machine in"=w4959) -> ("error out"=w4954:errorcluster, "State Machine out"=w4955:refnum<class "State Machine.lvclass">)  [unwired: 7 in]
          n1771 = call-dynamic "Write Timer.vi"("error in (no error)"=w4954, "Timer"=u32 40, "State Machine in"=w4955) -> ("error out"=w4951:errorcluster, "State Machine out"=w4952:refnum<class "State Machine.lvclass">)  [unwired: 7 in]
          n1772 = call-dynamic "Init Ticks2.vi"("error in (no error)"=w4951, "State Machine in"=w4952) -> ("error out"=w4950:errorcluster, "State Machine out"=w4949:refnum<class "State Machine.lvclass">)  [unwired: 8 in]
          n1773 = call-dynamic "Write State Machine.vi"("error in (no error)"=w4950, "State Machine.lvclass"=w4949, "Device in"=w4956) -> ("error out"=w4964:errorcluster, "Device out"=w4966:refnum<class "SecMirror.lvclass">)  [unwired: 7 in]
          n1774 = call-dynamic "Write SecMirror.lvclass.vi"("error in (no error)"=w4964, "SecMirror.lvclass"=w4966, "TelFocus in"=w4965) -> ("error out"=w4968:errorcluster, "TelFocus out"=w4967:refnum<class "TelFocus.lvclass">)  [unwired: 7 in]
          n1775 = call-dynamic "Write TelFocus.lvclass.vi"("error in (no error)"=w4968, "TelFocus.lvclass"=w4967, "S4GUI in"=w4975) -> ("error out"=w4973:errorcluster, "S4GUI out"=w4972:refnum<class "S4GUI.lvclass">)  [unwired: 7 in]
          n1776 = Increment(x=w4971) -> (x+1=w4970:u32)
          n1777 = Bundle By Name(cluster=w4972, "Obs_state"=w4970, "cyclesDone"=w4946, "sequesDone"=w4946) -> (w4969:refnum<class "S4GUI.lvclass">)
        }
        frame 361 {
          # "90: estado de erro."
          # "Timeout= 25s + distancia do target (cada 1000um=1s)"
          # "Espera terminar o movimento do foco do 2ndario para \ndisparar a aquisição do canal."
          n1778 = flat-sequence {
            tunnel: w5018 -> [w5040]
            tunnel: [w5040] -> w5017
            frame #0 {
              n1779 = Tick Count (ms)() -> (millisecond timer value=w5039:u32)
              "time 8" <- w5039
              n1780 = local read "time1"() -> (w5038:u32)
              n1781 = Subtract(x=w5039, y=w5038) -> (x-y=→"delay 78":u32)
            }
          }
          n1782 = call-dynamic "Read TelFocus.lvclass.vi"("error in (no error)"=w5017, "S4GUI in"=w5022) -> ("error out"=w5027:errorcluster, "TelFocus.lvclass"=w5028:refnum<class "TelFocus.lvclass">, "S4GUI out"=w5024:refnum<class "S4GUI.lvclass">)  [unwired: 7 in]
          n1783 = call-dynamic "Read SecMirror.lvclass.vi"("error in (no error)"=w5027, "TelFocus in"=w5028) -> ("error out"=w4996:errorcluster, "SecMirror.lvclass"=w4999:refnum<class "SecMirror.lvclass">, "TelFocus out"=w5026:refnum<class "TelFocus.lvclass">)  [unwired: 7 in]
          n1784 = call-dynamic "Read position.vi"("error in (no error)"=w4996, "SecMirror in"=w4999) -> ("error out"=w4995:errorcluster, "position"=w4992:i32, "SecMirror out"=w4998:refnum<class "SecMirror.lvclass">)  [unwired: 7 in]
          n1785 = call-dynamic "Read target.vi"("error in (no error)"=w4995, "SecMirror in"=w4998) -> ("error out"=w4994:errorcluster, "target"=w4993:i32, "SecMirror out"=w4997:refnum<class "SecMirror.lvclass">)  [unwired: 7 in]
          n1786 = Subtract(x=w4993, y=w4992) -> (x-y=w4991:i32)
          n1787 = Absolute Value(x=w4991) -> (abs(x)=w4990:i32)
          n1788 = call-dynamic "Read State Machine.vi"("error in (no error)"=w4994, "Device in"=w4997) -> ("error out"=w5007:errorcluster, "State Machine.lvclass"=w5010:refnum<class "State Machine.lvclass">, "Device out"=w5020:refnum<class "SecMirror.lvclass">)  [unwired: 7 in]
          n1789 = To Unsigned Long Integer(number=w4990) -> (unsigned 32bit integer=w4987:u32)
          n1790 = Add(x=w4987, y=u32 25000 ("period")) -> (x+y=w4988:u32)
          n1791 = call-dynamic "Verif Clock 2.vi"("error in (no error)"=w5007, "period (ms)"=w4988, "State Machine in"=w5010) -> ("error out"=w5006:errorcluster, "time elapsed"=→"time elapsed 2":u32, "State Machine out"=w5009:refnum<class "State Machine.lvclass">)  [unwired: 6 in]
          n1792 = call-dynamic "Read Timeout 2.vi"("error in (no error)"=w5006, "State Machine in"=w5009) -> ("error out"=w5005:errorcluster, "Timeout 2"=w4983:bool, "State Machine out"=w5008:refnum<class "State Machine.lvclass">)  [unwired: 7 in]
          n1793 = call-dynamic "Read State.vi"("error in (no error)"=w5005, "State Machine in"=w5008) -> ("error out"=w5015:errorcluster, "State"=w4986:i32, "State Machine out"=w5016:refnum<class "State Machine.lvclass">)  [unwired: 7 in]
          n1794 = Equal To 0?(x=w4986) -> (x = 0?=w4981:bool)
          n1795 = Equal?(x=w4986, y=90) -> (x = y?=w4984:bool)
          n1796 = call-dynamic "Write State Machine.vi"("error in (no error)"=w5015, "State Machine.lvclass"=w5016, "Device in"=w5020) -> ("error out"=w5019:errorcluster, "Device out"=w5021:refnum<class "SecMirror.lvclass">)  [unwired: 7 in]
          n1797 = call-dynamic "Write SecMirror.lvclass.vi"("error in (no error)"=w5019, "SecMirror.lvclass"=w5021, "TelFocus in"=w5026) -> ("error out"=w5023:errorcluster, "TelFocus out"=w5025:refnum<class "TelFocus.lvclass">)  [unwired: 7 in]
          n1798 = Or(x=w4984, y=w4983) -> (x .or. y?=w4982:bool)
          n1799 = call-dynamic "Write TelFocus.lvclass.vi"("error in (no error)"=w5023, "TelFocus.lvclass"=w5025, "S4GUI in"=w5024) -> ("error out"=w5012:errorcluster, "S4GUI out"=w5004:refnum<class "S4GUI.lvclass">)  [unwired: 7 in]
          n1800 = case shown="False" w4982 {
            tunnel: w5011 -> [w5031 _]
            tunnel: [w5031 u32 1 ("Obs_state")] -> w5001
            tunnel: w5004 -> [w5030 w5036]
            tunnel: [w5030 w5035] -> w5003
            tunnel: [w5029 FALSE] -> w4980
            tunnel: w4981 -> [w5029 _]
            frame False {
            }
            frame True {
              n1801 = Bundle By Name(cluster=w5036, "Error Msg"="ERROR: moving telescope focus timeout  (S4GUI:HandleObservationSync.vi - state 361)") -> (w5035:refnum<class "S4GUI.lvclass">)
            }
          }
          n1802 = Increment(x=w5001) -> (x+1=w5000:u32)
          n1803 = Select(t=w5000, s=w4980, f=w5001) -> (s? t:f=w5014:u32)
          n1804 = Bundle By Name(cluster=w5003, "Obs_state"=w5014) -> (w5013:refnum<class "S4GUI.lvclass">)
        }
        frame 362 {
          # "Envia dados para o header das imagens (Channel:Run.vi - estado 58)"
          n1805 = call-dynamic "Read AcquisitionA.vi"("error in (no error)"=w5082, "S4ACS_GUI in"=w5083) -> ("error out"=w5059:errorcluster, "Acquisition.lvclass"=w5062:refnum<class "Acquisition.lvclass">, "S4ACS_GUI out"=w5085:refnum<class "S4GUI.lvclass">)  [unwired: 7 in]
          n1806 = call-dynamic "Read enabled.vi"("error in (no error)"=w5059, "Server in"=w5062) -> ("error out"=w5058:errorcluster, "enabled"=w5060:bool, "Server out"=w5061:refnum<class "Acquisition.lvclass">)  [unwired: 7 in]
          n1807 = case shown="True" w5060 {
            tunnel: w5061 -> [w5141 w5156]
            tunnel: w5058 -> [w5140 w5155]
            tunnel: [w5141 w5153] -> w5086
            tunnel: [w5140 w5152] -> w5084
            frame False {
            }
            frame True {
              n1808 = call-dynamic "Read Channel.vi"("error in (no error)"=w5155, "Acquisition in"=w5156) -> ("error out"=w5148:errorcluster, "Channel.lvclass"=w5147:refnum<class "Channel.lvclass">, "Acquisition out"=w5154:refnum<class "Acquisition.lvclass">)  [unwired: 7 in]
              n1809 = call-dynamic "Read State Machine.vi"("error in (no error)"=w5148, "Device in"=w5147) -> ("error out"=w5149:errorcluster, "State Machine.lvclass"=w5151:refnum<class "State Machine.lvclass">, "Device out"=w5145:refnum<class "Channel.lvclass">)  [unwired: 7 in]
              n1810 = call "Next State.vi"("error in (no error)"=w5149, "New_State"=58, "State Machine in"=w5151) -> ("error out"=w5142:errorcluster, "State Machine out"=w5143:refnum<class "State Machine.lvclass">)  [unwired: 7 in]
              n1811 = call-dynamic "Write State Machine.vi"("error in (no error)"=w5142, "State Machine.lvclass"=w5143, "Device in"=w5145) -> ("error out"=w5144:errorcluster, "Device out"=w5146:refnum<class "Channel.lvclass">)  [unwired: 7 in]
              n1812 = call-dynamic "Write Channel.vi"("error in (no error)"=w5144, "Channel.lvclass"=w5146, "Acquisition in"=w5154) -> ("error out"=w5152:errorcluster, "Acquisition out"=w5153:refnum<class "Acquisition.lvclass">)  [unwired: 7 in]
            }
          }
          n1813 = call-dynamic "Write AcquisitionA.vi"("error in (no error)"=w5084, "Acquisition.lvclass"=w5086, "S4ACS_GUI in"=w5085) -> ("error out"=w5077:errorcluster, "S4ACS_GUI out"=w5078:refnum<class "S4GUI.lvclass">)  [unwired: 7 in]
          n1814 = call "Read AcquisitionB.vi"("error in (no error)"=w5077, "S4ACS_GUI in"=w5078) -> ("error out"=w5055:errorcluster, "Acquisition.lvclass"=w5057:refnum<class "Acquisition.lvclass">, "S4ACS_GUI out"=w5075:refnum<class "S4GUI.lvclass">)  [unwired: 7 in]
          n1815 = call-dynamic "Read enabled.vi"("error in (no error)"=w5055, "Server in"=w5057) -> ("error out"=w5054:errorcluster, "enabled"=w5053:bool, "Server out"=w5056:refnum<class "Acquisition.lvclass">)  [unwired: 7 in]
          n1816 = case shown="True" w5053 {
            tunnel: w5056 -> [w5124 w5139]
            tunnel: w5054 -> [w5123 w5138]
            tunnel: [w5124 w5136] -> w5076
            tunnel: [w5123 w5135] -> w5074
            frame False {
            }
            frame True {
              n1817 = call-dynamic "Read Channel.vi"("error in (no error)"=w5138, "Acquisition in"=w5139) -> ("error out"=w5131:errorcluster, "Channel.lvclass"=w5130:refnum<class "Channel.lvclass">, "Acquisition out"=w5137:refnum<class "Acquisition.lvclass">)  [unwired: 7 in]
              n1818 = call-dynamic "Read State Machine.vi"("error in (no error)"=w5131, "Device in"=w5130) -> ("error out"=w5132:errorcluster, "State Machine.lvclass"=w5134:refnum<class "State Machine.lvclass">, "Device out"=w5128:refnum<class "Channel.lvclass">)  [unwired: 7 in]
              n1819 = call "Next State.vi"("error in (no error)"=w5132, "New_State"=58, "State Machine in"=w5134) -> ("error out"=w5125:errorcluster, "State Machine out"=w5126:refnum<class "State Machine.lvclass">)  [unwired: 7 in]
              n1820 = call-dynamic "Write State Machine.vi"("error in (no error)"=w5125, "State Machine.lvclass"=w5126, "Device in"=w5128) -> ("error out"=w5127:errorcluster, "Device out"=w5129:refnum<class "Channel.lvclass">)  [unwired: 7 in]
              n1821 = call-dynamic "Write Channel.vi"("error in (no error)"=w5127, "Channel.lvclass"=w5129, "Acquisition in"=w5137) -> ("error out"=w5135:errorcluster, "Acquisition out"=w5136:refnum<class "Acquisition.lvclass">)  [unwired: 7 in]
            }
          }
          n1822 = call "Write AcquisitionB.vi"("error in (no error)"=w5074, "Acquisition.lvclass"=w5076, "S4ACS_GUI in"=w5075) -> ("error out"=w5070:errorcluster, "S4ACS_GUI out"=w5069:refnum<class "S4GUI.lvclass">)  [unwired: 7 in]
          n1823 = call-dynamic "Read AcquisitionC.vi"("error in (no error)"=w5070, "S4ACS_GUI in"=w5069) -> ("error out"=w5050:errorcluster, "Acquisition.lvclass"=w5052:refnum<class "Acquisition.lvclass">, "S4ACS_GUI out"=w5072:refnum<class "S4GUI.lvclass">)  [unwired: 7 in]
